vi "Created Insert.vi"(9 "Created":refnum<user-event>, 10 "Created Alias":string, 11 "Base Addresses Strategy in":refnum<class "Base Addresses Strategy.lvclass">) -> (3 "Base Addresses Strategy out":refnum<class "Base Addresses Strategy.lvclass">)   [LabVIEW 2021, in "jettl.lvlib" / "Addresses Strategy.lvlib" / "Base Addresses Strategy.lvclass"]
uses:
  Base Addresses Strategy.lvclass
  Msg Strategy/Msg Strategy.lvclass
  Base Addresses Strategy.lvclass/Base Addresses Strategy.ctl
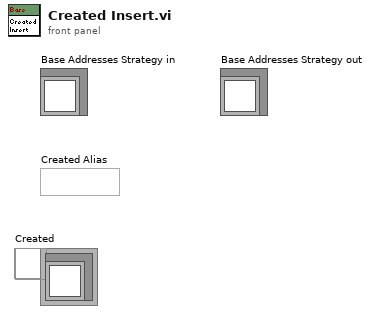
[diagram p1: front panel]
types:
  T1 = typedef "jettl.lvlib/Addresses Strategy.lvlib/Created.ctl" = map{string, refnum<user-event>}
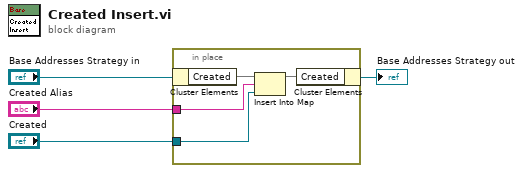
[diagram p0: block diagram]
diagram:
  n1 = in-place {
    in-place-border: "Created Alias" -> [w8]
    in-place-border: "Created" -> [w5]
    n2 = in-place-cluster #1("Base Addresses Strategy in") -> ("Created"=w7:T1)
    n3 = Insert Into Map(map in=w7, key=w8, value=w5) -> (map out=w6:T1)  [unwired: 2 out]
    n4 = in-place-cluster #1("Created"=w6) -> (→"Base Addresses Strategy out":refnum<class "Base Addresses Strategy.lvclass">)
  }
